vi "Unbundle Code Cluster.vi"(11 "Array of Cluster":T1(array[cluster])) -> (2 "Defines":string[](array[string]), 3 "Includes":string[](array[string]))   [LabVIEW 2014]
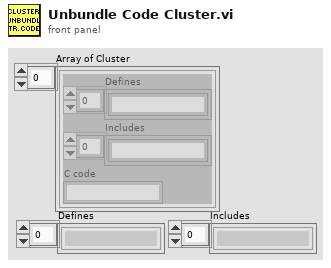
[diagram p1: front panel]
types:
  T1 = cluster{"Defines":string[], "Includes":string[], "C code":string}[]
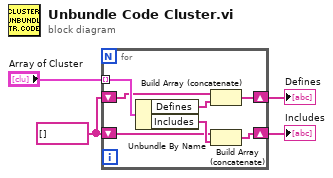
[diagram p0: block diagram]
diagram:
  w3 = string[] [] ("Defines")
  n1 = for {
    tunnel: "Array of Cluster" -> [w11] mode=indexing
    shift-right: [w9] -> w2
    shift-left: w3 -> [w8]
    shift-right: [w5] -> w1
    shift-left: w3 -> [w6]
    n2 = Unbundle By Name(w11) -> ("Defines"=w10:string[], "Includes"=w7:string[])
    n3 = Build Array (concatenate)(w8, w10) -> (w9:string[])
    n4 = Build Array (concatenate)(w6, w7) -> (w5:string[])
  }
  "Defines" <- w2
  "Includes" <- w1
